vi "Remove FPGA Sections.vi"(8 "error in (no error)":errorcluster, 11 "Item Ref in":T1 format="%.0x") -> (0 "error out":errorcluster, 3 "Item Ref out":T1 format="%.0x")   [LabVIEW 2015, in "Fuel Injector Analysis Addon System Explorer.lvlib"]
uses:
  Fuel Injector Analysis Addon System Explorer.lvlib
  <vilib>/NI Veristand/Custom Device API/Custom Device Item Ref.ctl
  <vilib>/NI Veristand/Custom Device Tools/Custom Device Utility Library/NI VeriStand - Search for All Items by GUID.vi
  Shared/Constants.vi
  <vilib>/NI VeriStand/Custom Device API/Custom Device API.lvlib
  <vilib>/NI Veristand/Custom Device Tools/Custom Device Utility Library/Custom Device Utility Library.lvlib
  Shared/Fuel Injector Analysis Addon Shared.lvlib
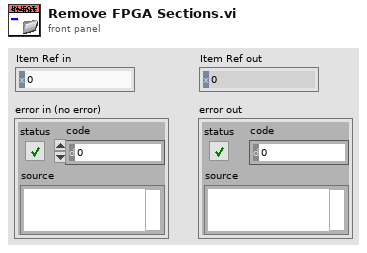
[diagram p1: front panel]
types:
  T1 = typedef "Custom Device API.lvlib/Custom Device Item Ref.ctl" = u64
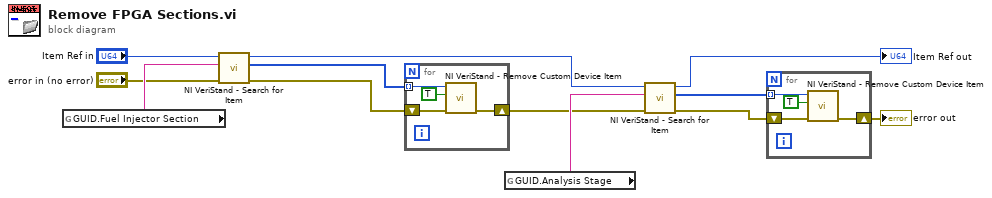
[diagram p0: block diagram]
diagram:
  n1 = global read "Constants.vi" "GUID.Fuel Injector Section"() -> (w12:string)
  n2 = call-poly <vilib>:"NI VeriStand - Search for Item.vi"("error in"="error in (no error)", "Item GUID"=w12, "Section Ref in"="Item Ref in") -> ("error out"=w11:errorcluster, "Item Refs"=w8:T1[], "Section Ref out"=w3:T1)  [unwired: 5 in, 1 out]
  n3 = for {
    tunnel: w8 -> [w16] mode=indexing
    shift-right: [w14] -> w4
    shift-left: w11 -> [w15]
    n4 = call <vilib>:"NI VeriStand - Remove Custom Device Item.vi"("error in (no error)"=w15, "Force Delete (F)"=TRUE, "Item Ref in"=w16) -> ("error out"=w14:errorcluster)  [unwired: 7 in, 1 out]
  }
  n5 = global read "Constants.vi" "GUID.Analysis Stage"() -> (w5:string)
  n6 = call-poly <vilib>:"NI VeriStand - Search for Item.vi"("error in"=w4, "Item GUID"=w5, "Section Ref in"=w3) -> ("error out"=w6:errorcluster, "Item Refs"=w7:T1[], "Section Ref out"=→"Item Ref out":T1)  [unwired: 5 in, 1 out]
  n7 = for {
    tunnel: w7 -> [w20] mode=indexing
    shift-right: [w18] -> w1
    shift-left: w6 -> [w19]
    n8 = call <vilib>:"NI VeriStand - Remove Custom Device Item.vi"("error in (no error)"=w19, "Force Delete (F)"=TRUE, "Item Ref in"=w20) -> ("error out"=w18:errorcluster)  [unwired: 7 in, 1 out]
  }
  "error out" <- w1
